vi "2D Arrays One Larger Than The Other.vi"() -> ()   [LabVIEW 2012]
uses:
  <vilib>/Analysis/Matrix/Numeric/Conversions/Array To Matrix - RA2.vi
  <vilib>/Analysis/baseanly.llb/Real A x B.vi
  <vilib>/Analysis/Matrix/Numeric/Conversions/Matrix To Array - RM.vi
  <vilib>/Analysis/NI_AALBase.lvlib
  <vilib>/Analysis/Matrix/NI_Matrix.lvlib
panel:
  out "Final Output  Array  (Original With Smaller * Sub)":dbl[][](array[numeric])
  out "Sub Array":dbl[][](array[numeric])
  in  "Original Smaller Array":dbl[][](array[numeric])
  in  "Original Larger Array":dbl[][](array[numeric])
  # "Enter Values Into The Arrays Below"
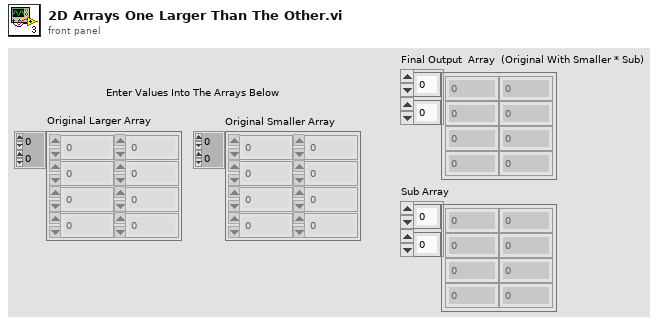
[diagram p1: front panel]
types:
  T1 = typedef "NI_Matrix.lvlib/RealMatrix.ctl" = dbl[][]
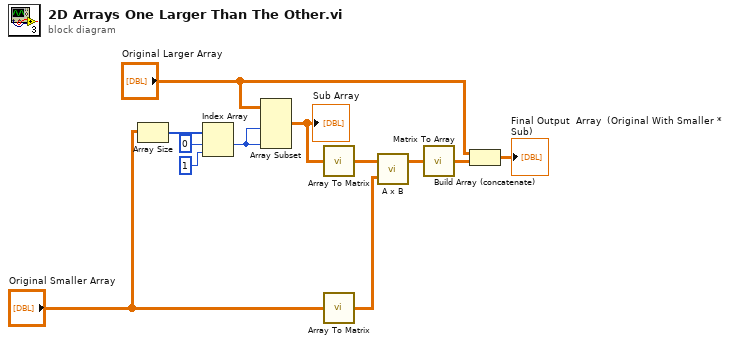
[diagram p0: block diagram]
diagram:
  n1 = Array Size(array="Original Smaller Array") -> (size(s)=w12:i32[])
  n2 = Index Array(array=w12, index #1=0 ("index"), index #2=1 ("index")) -> (element #1=w7:i32)  [unwired: 1 out]
  n3 = Array Subset(array="Original Larger Array", length (row)=w7, length (col)=w7) -> (w5:dbl[][])  [unwired: 2 in]
  "Sub Array" <- w5
  n4 = call-poly <vilib>:"Array To Matrix.vi"("Real 2D Array"=w5) -> ("Real Matrix"=w4:T1)
  n5 = call-poly <vilib>:"Array To Matrix.vi"("Real 2D Array"="Original Smaller Array") -> ("Real Matrix"=w3:T1)
  n6 = call-poly <vilib>:"A x B.vi"("B"=w3, "A"=w4) -> ("A x B"=w2:T1)  [unwired: 1 out]
  n7 = call-poly <vilib>:"Matrix To Array.vi"("Real Matrix"=w2) -> ("Real 2D Array"=w1:dbl[][])
  n8 = Build Array (concatenate)("Original Larger Array", w1) -> (→"Final Output  Array  (Original With Smaller * Sub)":dbl[][])
